vi "Read Indexes.vi"(11 "(WavIndex_Pointer)":refnum<class "WavIndex_Pointer.lvclass">) -> (2 "End Out":i32, 3 "Start Out":i32)   [LabVIEW 2020, in "WavIndex_Pointer.lvclass"]
uses:
  WavIndex_Pointer.lvclass
  WavIndex_Pointer.lvclass/WavIndex_Pointer.ctl
  Index_Pointer/Index_Pointer.lvclass
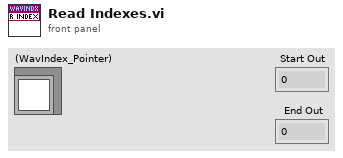
[diagram p1: front panel]
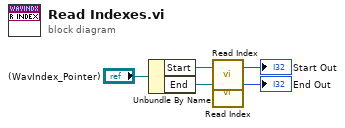
[diagram p0: block diagram]
diagram:
  n1 = Unbundle By Name("(WavIndex_Pointer)") -> ("Start"=w4:refnum<class "Index_Pointer.lvclass">, "End"=w3:refnum<class "Index_Pointer.lvclass">)
  n2 = call "Read Index.vi"("Index_Pointer)"=w4) -> ("Index Out"=→"Start Out":i32)  [unwired: 2 in]
  n3 = call "Read Index.vi"("Index_Pointer)"=w3) -> ("Index Out"=→"End Out":i32)  [unwired: 2 in]
